vi "All stations print config.vi"(10 "station idx":i32, 11 "configuration file path":path) -> (0 "error out":errorcluster caption="错误输出", 2 "station idx":i32, 3 "configuration file path":path, 5 "state prints config":T1)   [LabVIEW 2018]
uses:
  Crl defs/one state prints config.ctl
  Communication connection/Crl defs/print config.ctl
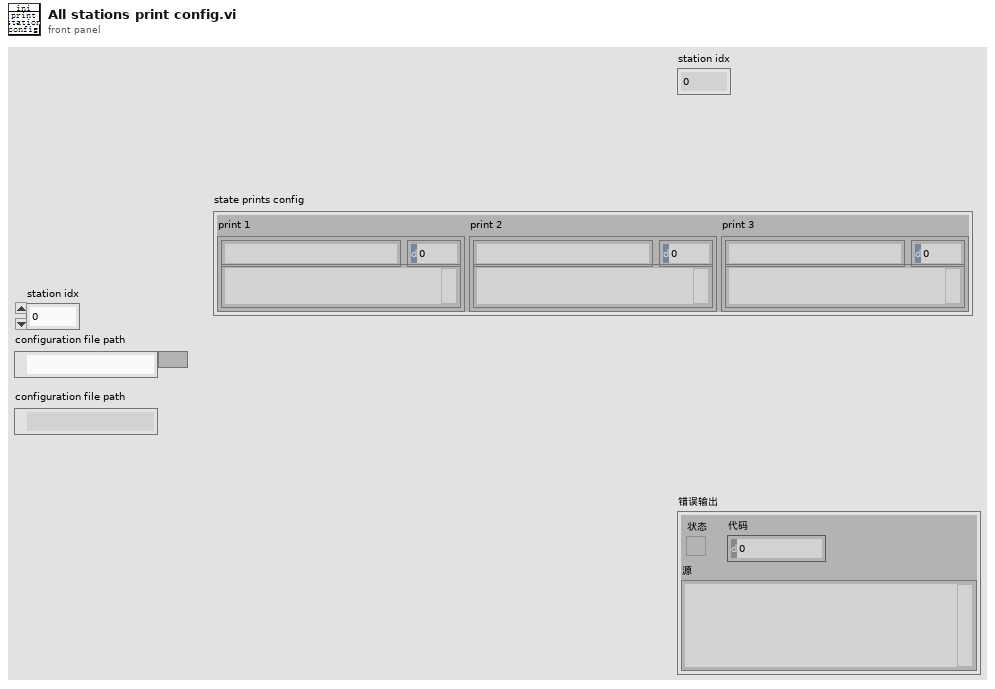
[diagram p1: front panel]
types:
  T1 = typedef "one state prints config.ctl" = cluster{"print 1":T2, "print 2":T2, "print 3":T2}
  T2 = typedef "print config.ctl" = cluster{"connect ip or coms":string, "port":u16, "print strings":string}
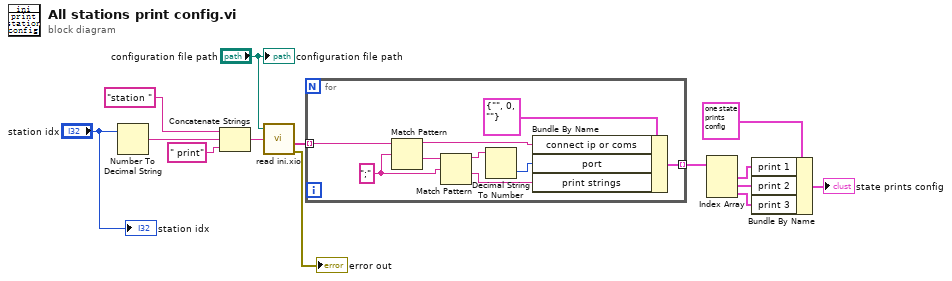
[diagram p0: block diagram]
diagram:
  n1 = Number To Decimal String(number="station idx") -> (decimal integer string=w14:string)  [unwired: 1 in]
  n2 = Concatenate Strings("station ", w14, " print" ("string")) -> (w11:string)
  n3 = call "read ini.xio.vi"("configuration file path"="configuration file path", "Sections"=w11) -> ("Values"=w8:string[], "error out"=→"error out":errorcluster)  [unwired: 1 in, 3 out]
  n4 = for {
    tunnel: w8 -> [w23] mode=indexing
    tunnel: [w15] -> w7 mode=indexing
    w21 = ";" ("正则表达式")
    n5 = Match Pattern(string=w23, regular expression=w21) -> (before substring=w19:string, after substring=w22:string)  [unwired: 1 in, 2 out]
    n6 = Match Pattern(string=w22, regular expression=w21) -> (before substring=w18:string, after substring=w16:string)  [unwired: 1 in, 2 out]
    n7 = Decimal String To Number(string=w18) -> (number=w17:i32)  [unwired: 2 in, 1 out]
    n8 = Bundle By Name(cluster=T2 {"connect ip or coms"="", "port"=0, "print strings"=""} ("print config"), "connect ip or coms"=w19, "port"=w17, "print strings"=w16) -> (w15:T2)
  }
  n9 = Index Array(array=w7) -> (element #1=w5:T2, element #2=w4:T2, element #3=w3:T2)  [unwired: 3 in]
  n10 = Bundle By Name(cluster=T1 {"print 1"={"connect ip or coms"="", "port"=0, "print strings"=""}, "print 2"={"connect ip or coms"="", "port"=0, "print strings"=""}, "print 3"={"connect ip or coms"="", "port"=0, "print strings"=""}} ("state prints config"), "print 1"=w5, "print 2"=w4, "print 3"=w3) -> (→"state prints config":T1)
  "configuration file path" <- "configuration file path"
  "station idx" <- "station idx"
